vi "Seed LVLIB.vi"(10 "Output Dir":path=path "C:/Test", 11 "LVLib Template Path":path) -> (2 "New LVLib":refnum<vi>)   [LabVIEW 2013]
panel:
  out "DEBUG Template Lib Name":string
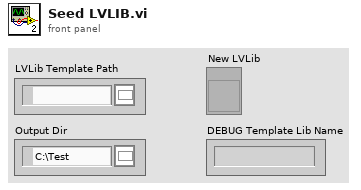
[diagram p1: front panel]
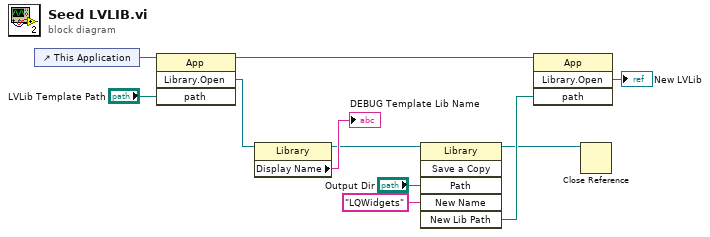
[diagram p0: block diagram]
diagram:
  n1 = control-ref of="This Application"() -> (w2:refnum<vi>)
  n2 = invoke class="App" method="Library.Open"(reference=w2, "path"="LVLib Template Path") -> (reference out=w8:refnum<vi>, "Open Library"=w11:refnum<vi>)  [unwired: 2 in, 2 out]
  n3 = property class="Library"(reference=w11) -> (reference out=w9:refnum<vi>, "Display Name"=→"DEBUG Template Lib Name":string)  [unwired: 1 in, 1 out]
  n4 = invoke class="Library" method="Save a Copy"(reference=w9, "Path"="Output Dir", "New Name"="LQWidgets") -> (reference out=w3:refnum<vi>, "New Lib Path"=w7:path)  [unwired: 3 in, 4 out]
  n5 = invoke class="App" method="Library.Open"(reference=w8, "path"=w7) -> ("Open Library"=→"New LVLib":refnum<vi>)  [unwired: 2 in, 3 out]
  n6 = Close Reference(reference=w3) -> ()  [unwired: 1 in, 1 out]
